vi "_FPGA_Driver_LTC1667_2.vi"(8 "Clk":bool, 10 "Data_in":fxp<+,14,14>) -> ()   [LabVIEW 2018]
uses:
  <vilib>/rvi/eio/common/nirviEmuTemplateMethod_errors.vi
  <vilib>/eio/EIONode/EIONode.xnode
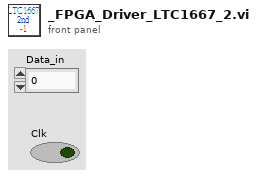
[diagram p1: front panel]
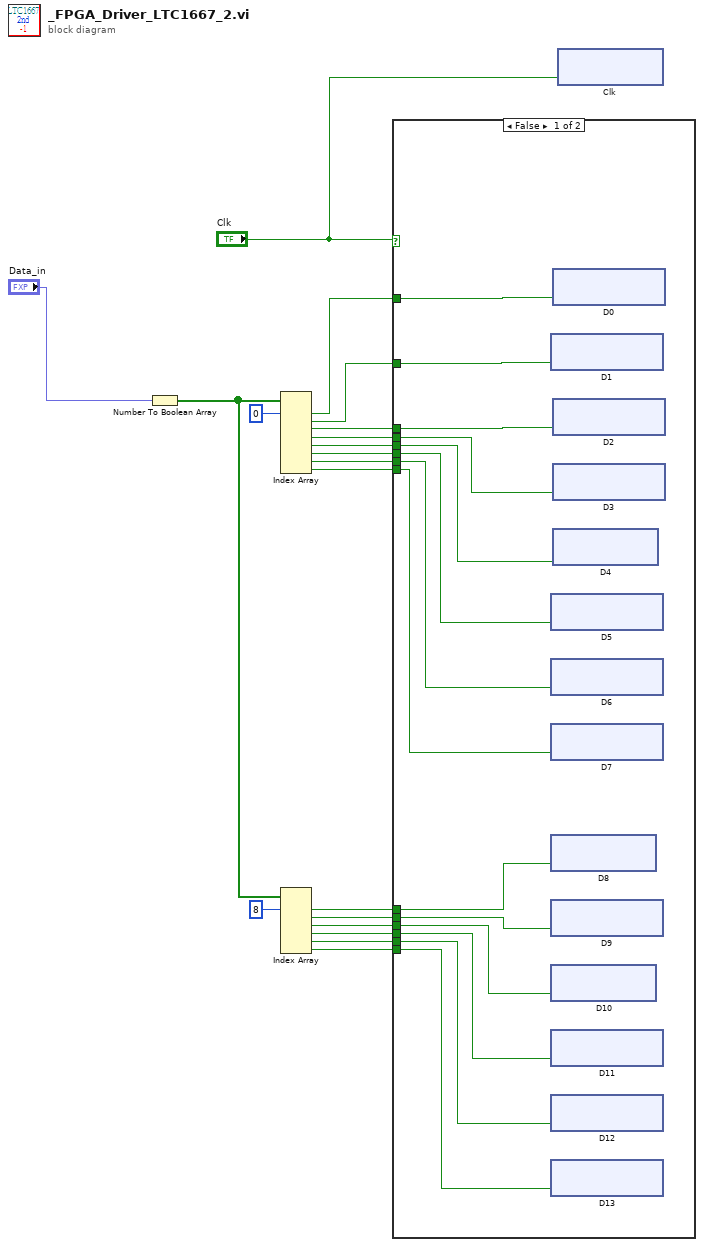
[diagram p0: block diagram]
diagram:
  n1 = Number To Boolean Array(number="Data_in") -> (Boolean array=w10:bool[])
  n2 = Index Array(array=w10, index #1=0 ("index")) -> (element #1=w18:bool, element #2=w17:bool, element #3=w16:bool, element #4=w15:bool, element #5=w14:bool, element #6=w13:bool, element #7=w12:bool, element #8=w11:bool)  [unwired: 7 in]
  n3 = Index Array(array=w10, index #1=8 ("index")) -> (element #1=w8:bool, element #2=w7:bool, element #3=w6:bool, element #4=w5:bool, element #5=w4:bool, element #6=w3:bool)  [unwired: 5 in]
  n4 = case shown="False" "Clk" {
    tunnel: w18 -> [w33 _]
    tunnel: w17 -> [w32 _]
    tunnel: w16 -> [w31 _]
    tunnel: w15 -> [w30 _]
    tunnel: w14 -> [w29 _]
    tunnel: w13 -> [w28 _]
    tunnel: w12 -> [w27 _]
    tunnel: w11 -> [w26 _]
    tunnel: w8 -> [w25 _]
    tunnel: w7 -> [w24 _]
    tunnel: w6 -> [w23 _]
    tunnel: w5 -> [w22 _]
    tunnel: w4 -> [w21 _]
    tunnel: w3 -> [w20 _]
    frame False {
      n5 = xnode "D1"("RMC/DIO74"=w32) -> ()  [unwired: 1 in, 1 out]
      n6 = xnode "D5"("RMC/DIO73"=w28) -> ()  [unwired: 1 in, 1 out]
      n7 = xnode "D6"("RMC/DIO40"=w27) -> ()  [unwired: 1 in, 1 out]
      n8 = xnode "D7"("RMC/DIO72"=w26) -> ()  [unwired: 1 in, 1 out]
      n9 = xnode "D8"("RMC/DIO8"=w25) -> ()  [unwired: 1 in, 1 out]
      n10 = xnode "D9"("RMC/DIO39"=w24) -> ()  [unwired: 1 in, 1 out]
      n11 = xnode "D10"("RMC/DIO7"=w23) -> ()  [unwired: 1 in, 1 out]
      n12 = xnode "D11"("RMC/DIO71"=w22) -> ()  [unwired: 1 in, 1 out]
      n13 = xnode "D12"("RMC/DIO38"=w21) -> ()  [unwired: 1 in, 1 out]
      n14 = xnode "D13"("RMC/DIO70"=w20) -> ()  [unwired: 1 in, 1 out]
      n15 = xnode "D0"("RMC/DIO42"=w33) -> ()  [unwired: 1 in, 1 out]
      n16 = xnode "D2"("RMC/DIO10"=w31) -> ()  [unwired: 1 in, 1 out]
      n17 = xnode "D3"("RMC/DIO41"=w30) -> ()  [unwired: 1 in, 1 out]
      n18 = xnode "D4"("RMC/DIO9"=w29) -> ()  [unwired: 1 in, 1 out]
    }
    frame True {
    }
  }
  n19 = xnode "Clk"("RMC/DIO6"="Clk") -> ()  [unwired: 1 in, 1 out]
